vi "Dashboard Main.vi"() -> ()   [LabVIEW 2015]
uses:
  <vilib>/Utility/miscctls.llb/LVRowAndColumnTypeDef.ctl
  <vilib>/event_ctls.llb/eventvkey.ctl
  <vilib>/Rock Robotics/WPI/Dashboard/WPI_DashboardLogging Global.vi
  <vilib>/Rock Robotics/Network Tables/NT Read Numeric Array.vi
  <vilib>/Rock Robotics/Network Tables/NT Write String Array.vi
  <vilib>/Rock Robotics/Network Tables/NT Write Numeric Array.vi
  <vilib>/Utility/config.llb/Write Key (String).vi
  <vilib>/Utility/config.llb/Write Key (I32).vi
  <vilib>/Utility/config.llb/NI_LVConfig.lvlib
panel:
  in  "TCP":refnum<k5>
  in  "Rec Mode":enum32{"Stop", "Record", "Playback"}(radio)
  in  "Vision":u16(ring) items=["Camera Off", "USB Camera SW", "USB Camera HW", "IP Camera"]
  out "Camera IP":string
  out "Image Message":string="Timeout in Camera Communications"
  in  "Dashboard Tab":T1(tab)
  in  "Auto Routines":string(combo)
  out "NT Connected":bool
  in  "Camera Settings":T2={"Frame Rate"=30, "Compression"=30, "Size"=1} {"Frame Rate" scale=1.0..30.0; "Size" items=["640x480", "320x240", "160x120"]}
  out "MotorChart R":cluster{"Numeric":dbl, "Numeric":dbl}(graph)
  out "MotorChart L":T3(graph)
  out "MotorSliders R":cluster{"MotorSlide1":dbl, "MotorSlide2":dbl} {"MotorSlide2" scale=-1.0..1.0 scale format="%#_2e"; "MotorSlide1" scale=-1.0..1.0 scale format="%#_2e"}
  out "MotorSliders L":T4 {"MotorSlide4 2" scale=0.0..14.0 scale format="%#_2e"; "MotorSlide2" scale=-1.0..1.0 scale format="%#_2e"; "MotorSlide1" scale=-1.0..1.0 scale format="%#_2e"}
  out "Gyro":dbl(knob) scale=0.0..360.0
  out "JS1 Z":dbl(slide) scale=-1.0..1.0 scale format="%#_2e"
  out "JS1 Graph":cluster{"X":dbl, "Y":dbl}[](graph)
  out "JS1 Buttons":T5
  out "JS2 Z":dbl(slide) scale=-1.0..1.0 scale format="%#_2e"
  out "JS2 Graph":cluster{"X":dbl, "Y":dbl}[](graph)
  out "JS2 Buttons":T5
  out "Mode":T6(ring)=enum."Auto Disabled"
  in  "DB Camera Config":bool
  out "fps":dbl format="%#.1g"
  out "Mbps":dbl format="%#.1g"
  out "Mbps 2":bool
  in  "DB/String 9":string
  in  "DB/String 8":string
  in  "DB/String 7":string
  in  "DB/String 6":string
  in  "DB/String 5":string
  in  "DB/String 4":string
  in  "DB/String 3":string
  in  "DB/String 2":string
  in  "DB/String 1":string
  in  "DB/String 0":string
  in  "DB/Slider 0":dbl(slide) scale=0.0..5.0
  in  "DB/Slider 1":dbl(slide) scale=0.0..5.0
  in  "DB/Slider 2":dbl(slide) scale=0.0..5.0
  in  "DB/Slider 3":dbl(slide) scale=0.0..5.0
  out "DB/LED 3":bool
  out "DB/LED 2":bool
  out "DB/LED 1":bool
  out "DB/LED 0":bool
  in  "DB/Button 3":bool
  in  "DB/Button 2":bool
  in  "DB/Button 1":bool
  in  "DB/Button 0":bool caption="New Name"
  in  "Test Slider":dbl(slide) scale=0.0..100.0 scale format="%#_3g"
  in  "On/Off":bool caption="Solenoid"
  in  "Test Name":u16(ring) items=["Select the test to run..."]
  in  "Test Tree":string(tree)
  in  "Motor":cluster{"Value":dbl, "Enable":bool} {"Value" scale=-1.0..1.0 scale format="%#_3g"}
  out "Progress":T7 {"Test Progress" scale=0.0..100.0}
  in  "Rev/Fwd":cluster{"Forward":bool, "Reverse":bool}
  in  "Test Ring":u16(ring) items=["Monochrome", "Color"]
  out "Cmd Status":string
  in  "Execute Command":bool
  in  "Command Params":string[][](table)
  in  "Command Selection":i32(listbox)
  in  "CheckList":i32(listbox)
  out "Tree":string(tree)
  out "Camera Image":T8(plugin-control)
  out "Boolean":bool
  # "Left"
  # "Front"
  # "Right"
  # "Battery"
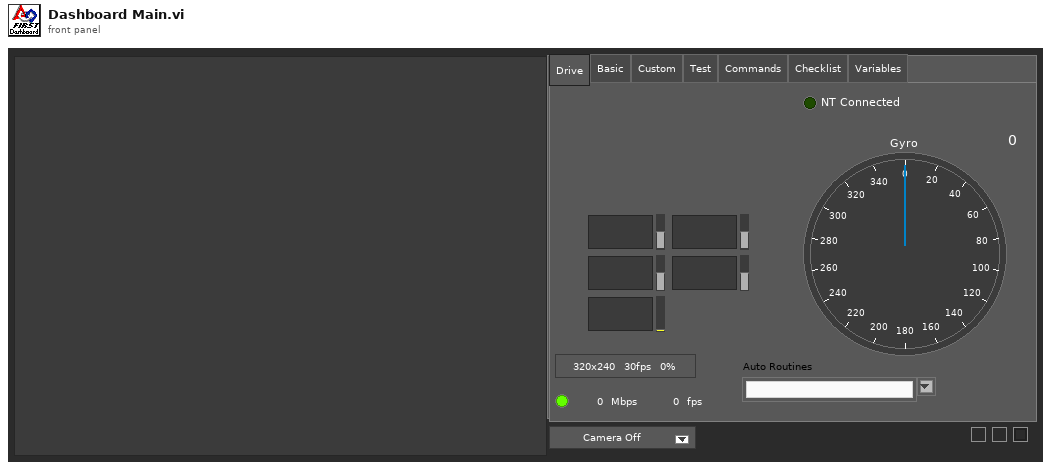
[diagram p1: front panel]
types:
  T1 = enum32{"Drive", "Basic", "Custom", "Test", "Commands", "Checklist", "Variables"}
  T2 = cluster{"Frame Rate":i32, "Compression":i32, "Size":u16}
  T3 = cluster{"Numeric":dbl, "Numeric":dbl, "Battery V":dbl}
  T4 = cluster{"MotorSlide1":dbl, "MotorSlide2":dbl, "MotorSlide4 2":dbl}
  T5 = cluster{bool, bool, bool, bool, bool, bool, bool, bool, bool, bool, bool, bool}
  T6 = enum8{"Tele-Op Disabled", "Tele-Op Enabled", "Auto Disabled", "Auto Enabled", "Test Disabled", "Test Enabled", "Disconnected", "No Code", "E-Stop"}
  T7 = cluster{"Test Progress":u8, "Test Progress Text":string}
  T8 = typedef "IMAQ Image.ctl" = refnum<image>
  T9 = cluster{"IDs":cluster{"RPC field ID":u16, "Unique ID":u16}, "String":string}
  T10 = enum32{"Drive", "Basic", "Custom", "Test", "Checklist", "Variables"}
  T11 = typedef "Image Type" = u32
  T12 = cluster{"Camera Image":refnum<vi>, "Dashboard Tab":refnum<vi>, "Boolean":refnum<vi>, "Vision":refnum<vi>, "Rec Mode":refnum<vi>, "Test Slider":refnum<vi>, "On/Off ":refnum<vi>, "Test Ring":refnum<vi>, "Rev/Fwd":refnum<vi>, "Test Name":refnum<vi>, "Motor":refnum<vi>, "Progress":refnum<vi>, "CheckList":refnum<vi>, "Tree":refnum<vi>, "Test Tree":refnum<vi>, "Command Params":refnum<vi>, "Command Selection":refnum<vi>, "Execute Command":refnum<vi>, "Cmd Status":refnum<vi>}
  T13 = cluster{"Error Strings":string, "Disable Counts":cluster{u16, u16}, "Rail Faults":cluster{u16, u16, u16}, "Robot IP":string, "DB Mode":u8, "Event Info":cluster{"Name":string, "Type":u8, "Number":u16, "Replay":u8}, "Camera Addr":string}
  T14 = cluster{"Storage":cluster{"Disk Free":u64, "RAM Block":u32, "RAM free":u32}, "CPU Utilization":cluster{"CPU % ISR":sgl, "CPU % Time Crit":sgl, "CPU % Timed Str":sgl, "CPU % High":sgl, "CPU % Above":sgl, "CPU % Normal":sgl, "CPU % Low":sgl}, "CAN":cluster{"% Bus Utilization":sgl, "Bus Off Cnt":u32, "TX_FIFO Full Cnt":u32, "Receive Error Cnt":u8, "Transmit Error Cnt":u8}, "HID":cluster{"HID Outputs":u32, "Rumble Low":u16, "Rumble High":u16}[]}
  T15 = cluster{"Status bits":cluster{"Test Mode":bool, "Autonomous":bool, "Enabled":bool, "Code Start":bool, "Brownout":bool, "Reserved 2":bool, "Reserved 3":bool, "E-Stop":bool}, "Code Trace":cluster{"Disabled":bool, "TeleOp":bool, "Auto":bool, "Test":bool}, "Controller Type":enum16{"unknown", "cRIO", "roboRio"}, "Code?":enum16{"unknown", "noCode", "code"}, "Battery V":dbl}
  T16 = cluster{"Control Bits":cluster{"TestMode":bool, "Autonomous":bool, "Enabled":bool, "FMS Present":bool, bool, bool, bool, "E-Stop":bool}, "Team Station ":u8, "Countdown":sgl, "Joystick Values":cluster{"Axes":dbl[], "Buttons":bool[], "POVs":i16[]}[]}
  T17 = cluster{"Axes":dbl[], "Buttons":bool[], "POVs":i16[]}[]
  T18 = cluster{"Axes":dbl[], "Buttons":bool[], "POVs":i16[]}
  T19 = cluster{"Buttons[0]":bool, "Buttons[1]":bool, "Buttons[2]":bool, "Buttons[3]":bool, "Buttons[4]":bool, "Buttons[5]":bool, "Buttons[6]":bool, "Buttons[7]":bool, "Buttons[8]":bool, "Buttons[9]":bool, "Buttons[10]":bool, "Buttons[11]":bool}
  T20 = typedef "NI_LVConfig.lvlib/Config Data RefNum.ctl" = refnum<k1>
  T21 = cluster{"Operation":enum16{"Update", "Clear"}, "Color Box":u32}[]
  T22 = typedef "eventvkey.ctl" = enum16{"ASCII", "Enter", "Return", "Shift", "Ctrl", "Alt", "Cmd", "Opt", "Caps", "NumLock", "Clear", "Break", "Up", "Down", "Left", "Right", "Insert", "Delete", "Home", "End", "PageUp", "PageDown", "Escape", "Help", "Pause", "ScrollLock", "F1", "F2", "F3", "F4", "F5", "F6", "F7", "F8", "F9", "F10", "F11", "F12", "F13", "F14", "F15", "F16", "F17", "F18", "F19", "F20", "F21", "F22", "F23", "F24", "Play", "VolumeUp", "VolumeDown", "Mute", "Two Byte Char"}
  T23 = cluster{"Image Size":bool, "Image Type":bool, "Pixel Value":bool, "ROI Information":bool, "Zoom Factor":bool}
  T24 = enum8{"Enabled", "Disabled", "Disabled and Grayed Out"}
  T25 = cluster{"Operation":enum16{"Update", "Clear"}, "Color Box":u32}
  T26 = typedef "LVRowAndColumnTypeDef.ctl" = cluster{"Row":i32, "Column":i32}
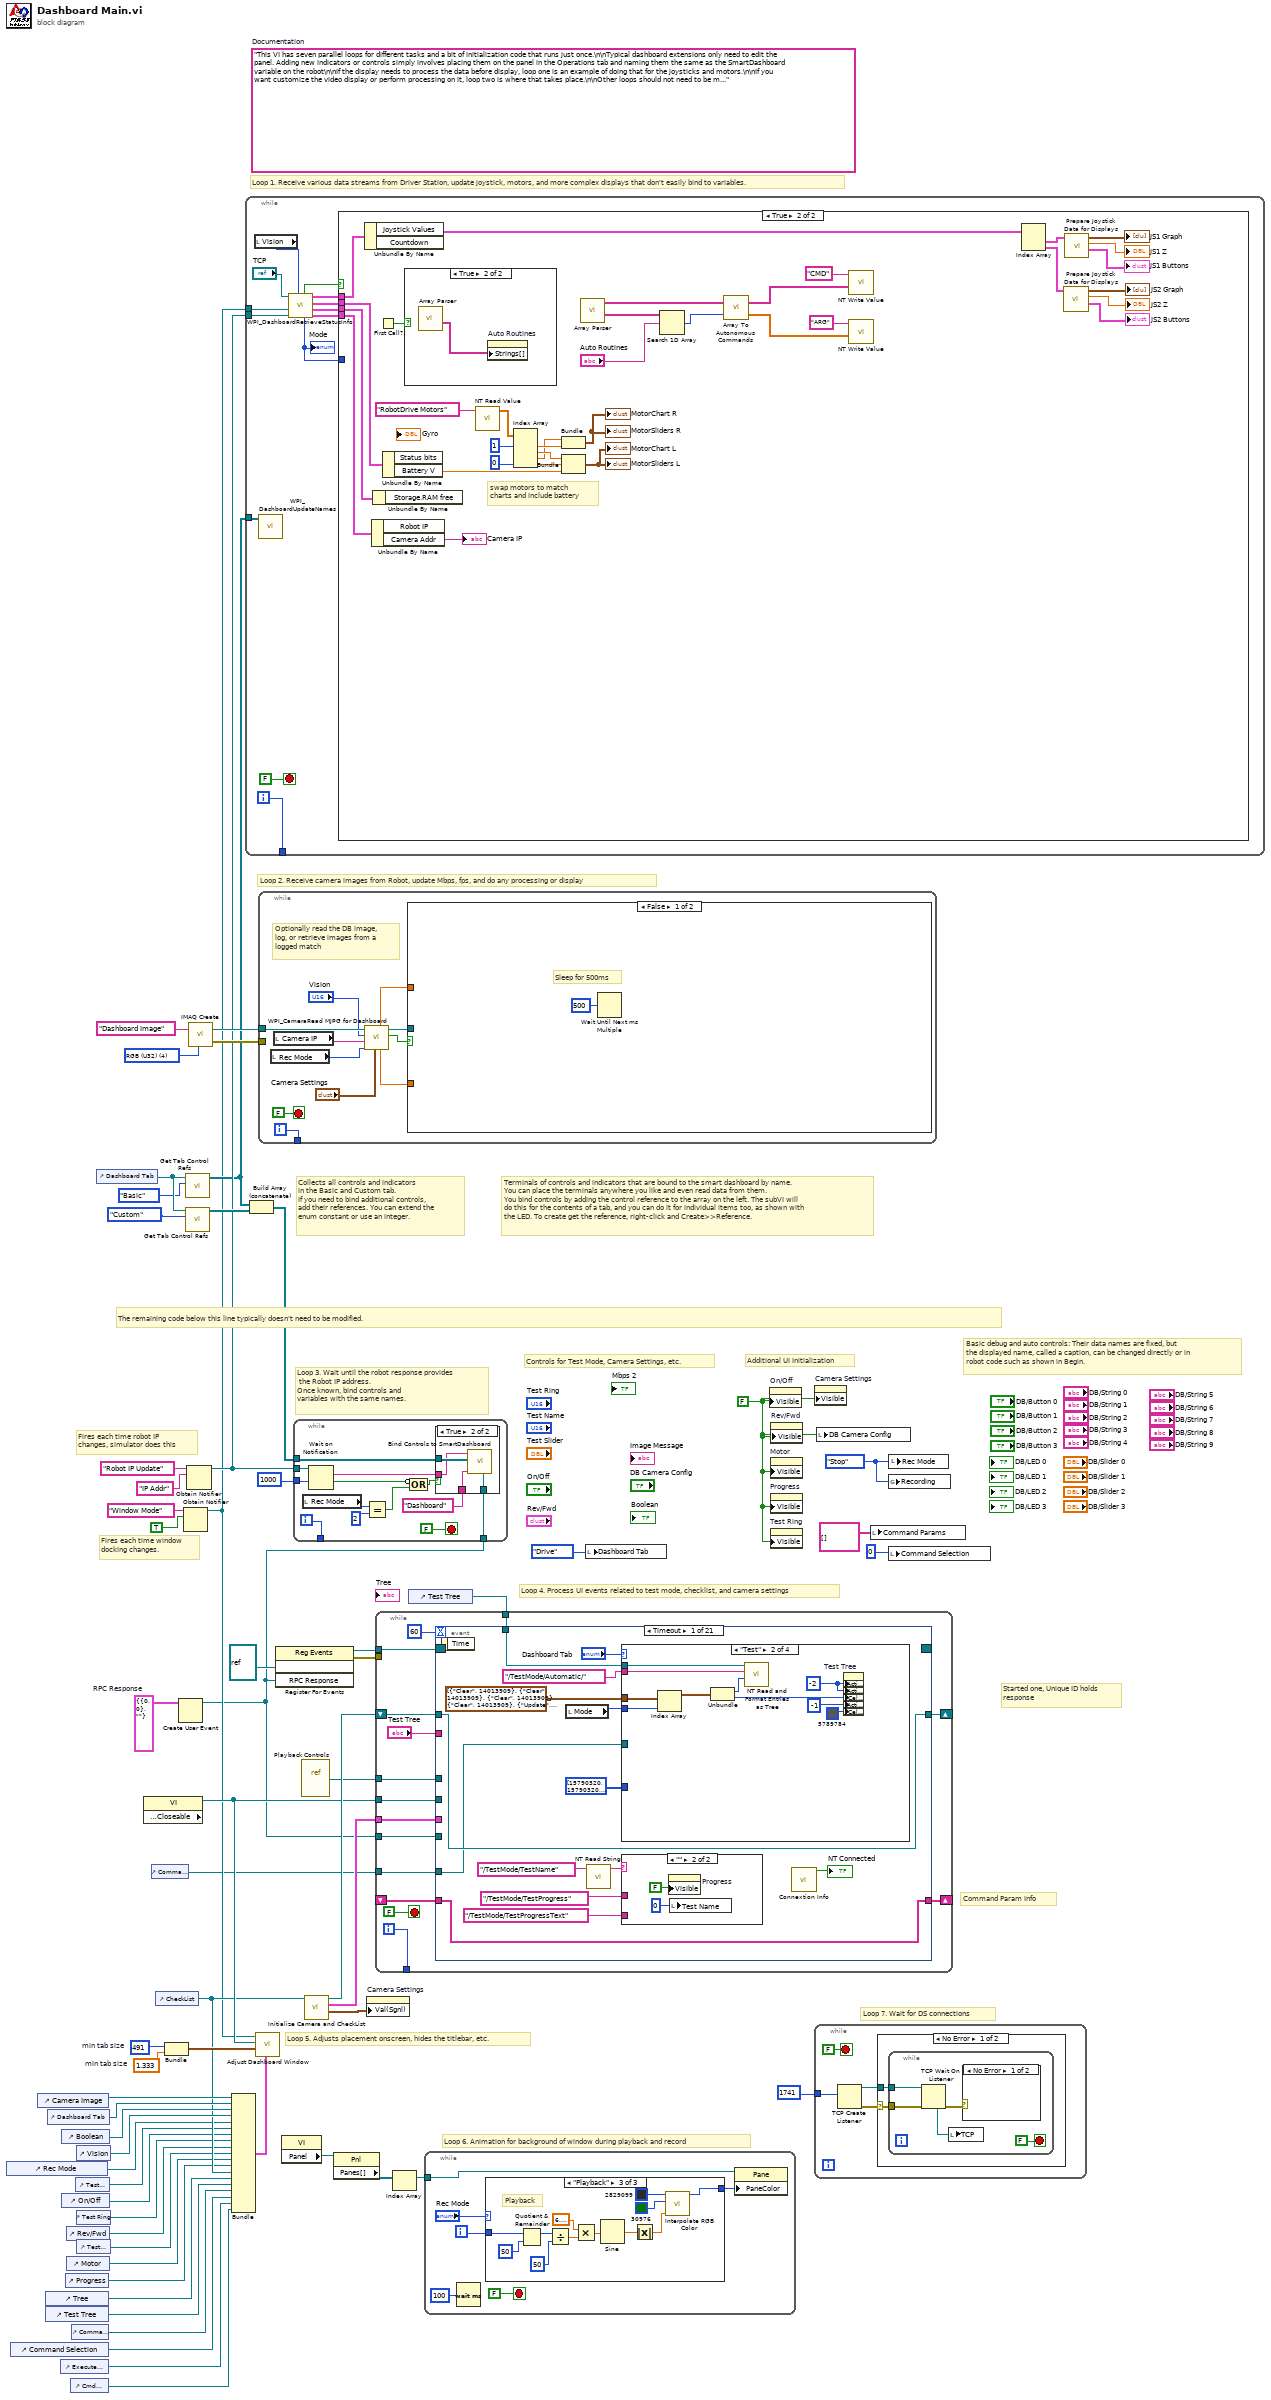
[diagram p0: block diagram]
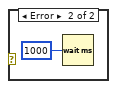
[diagram p2: hidden frame]
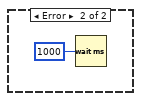
[diagram p3: hidden frame]
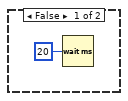
[diagram p4: hidden frame]
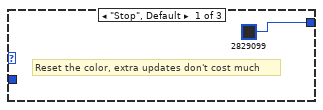
[diagram p6: hidden frame]
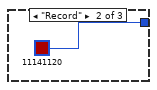
[diagram p7: hidden frame]
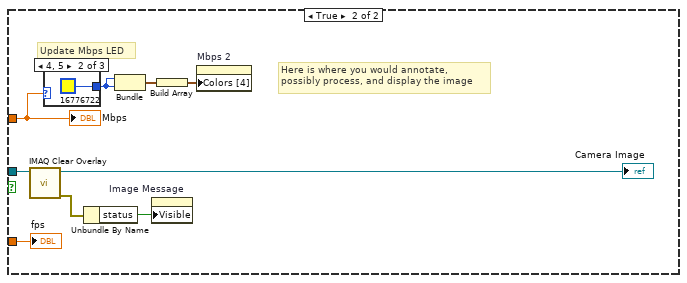
[diagram p9: hidden frame]
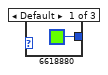
[diagram p10: hidden frame]
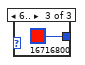
[diagram p11: hidden frame]
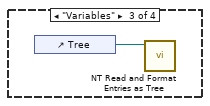
[diagram p13: hidden frame]
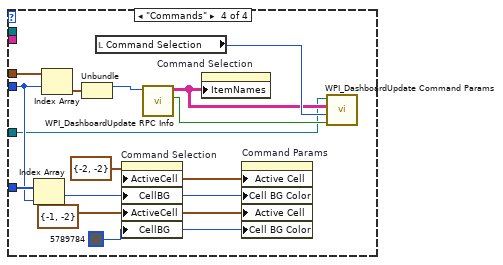
[diagram p14: hidden frame]
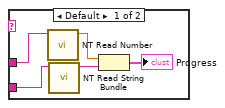
[diagram p15: hidden frame]
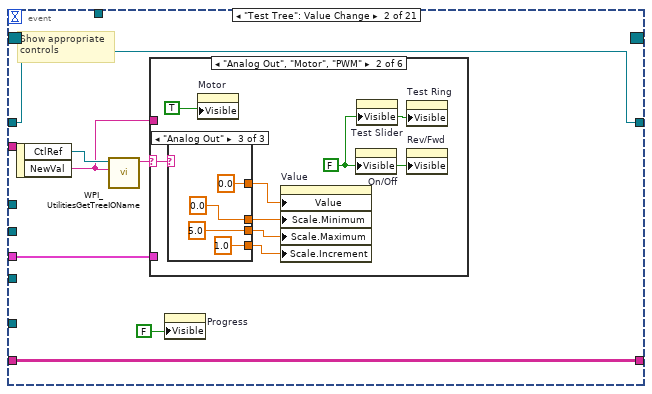
[diagram p16: hidden frame]
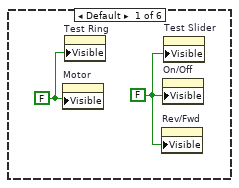
[diagram p17: hidden frame]
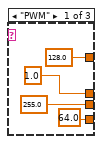
[diagram p18: hidden frame]
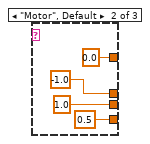
[diagram p19: hidden frame]
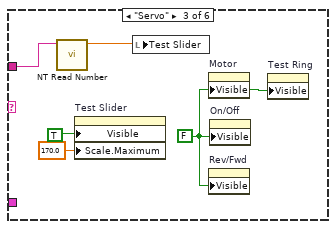
[diagram p20: hidden frame]
diagram:
  w7 = T9 {"IDs"={"RPC field ID"=0, "Unique ID"=0}, "String"=""}  # RPC Response
  w33 = 491  # min tab size
  w32 = 1.333  # min tab size
  w41 = enum32{"Stop", "Record", "Playback"}."Stop" ("Rec Mode")
  w15 = FALSE ("Visible")
  (unwired) "This VI has seven parallel loops for different tasks and a bit of initialization code that runs just once.\n\nTypical dashboard extensions only need to edit the panel. Adding new indicators or controls simply involves placing them on the panel in the Operations tab and naming them the same as the SmartDashboard variable on the robot\n\nIf the display needs to process the data before display, loop one is an example of doing that for the joysticks and motors.\n\nIf you want customize the video display or perform processing on it, loop two is where that takes place.\n\nOther loops should not need to be modified. They are pretty standard, and document the task they perform."  # Documentation
  w61 = T11 4 items=["Grayscale (U8)", "Grayscale (I16)", "Grayscale (SGL)", "Complex (CSG)", "RGB (U32)", "HSL (U32)", "RGB (U64)"] ("Image Type")
  # "Command Param Info"
  # "Started one, Unique ID holds\nresponse"
  # "Loop 7. Wait for DS connections"
  # "Basic debug and auto controls: Their data names are fixed, but\nthe displayed name, called a caption, can be changed directly or in\nrobot code such as shown in Begin."
  # "Controls for Test Mode, Camera Settings, etc."
  # "Additional UI Initialization"
  # "Loop 6. Animation for background of window during playback and record"
  # "Fires each time robot IP\nchanges, simulator does this"
  # "Fires each time window\ndocking changes."
  # "Collects all controls and indicators\nin the Basic and Custom tab.\nIf you need to bind additional controls,\nadd their references. You can extend the\nenum constant or use an integer."
  # "The remaining code below this line typically doesn't need to be modified."
  # "Loop 4. Process UI events related to test mode, checklist, and camera settings"
  # "Terminals of controls and indicators that are bound to the smart dashboard by name.\nYou can place the terminals anywhere you like and even read data from them.\nYou bind controls by adding the control reference to the array on the left. The subVI will\ndo this for the contents of a tab, and you can do it for individual items too, as shown with\nthe LED. To create get the reference, right-click and Create>>Reference."
  # "Loop 3. Wait until the robot response provides\n the Robot IP address.\nOnce known, bind controls and\nvariables with the same names."
  # "Loop 5. Adjusts placement onscreen, hides the titlebar, etc."
  # "Loop 1. Receive various data streams from Driver Station, update joystick, motors, and more complex displays that don't easily bind to variables."
  # "Loop 2. Receive camera images from Robot, update Mbps, fps, and do any processing or display"
  n1 = control-ref of="Rec Mode"() -> (w21:refnum<vi>)
  n2 = control-ref of="Command Selection"() -> (w6:refnum<vi>)
  n3 = control-ref of="Camera Image"() -> (w36:refnum<vi>)
  n4 = control-ref of="Tree"() -> (w25:refnum<vi>)
  n5 = control-ref of="Test Tree"() -> (w24:refnum<vi>)
  n6 = control-ref of="Dashboard Tab"() -> (w35:refnum<vi>)
  n7 = control-ref of="Execute Command"() -> (w8:refnum<vi>)
  n8 = control-ref of="Boolean"() -> (w30:refnum<vi>)
  n9 = control-ref of="On/Off"() -> (w19:refnum<vi>)
  n10 = control-ref of="Progress"() -> (w16:refnum<vi>)
  n11 = control-ref of="Rev/Fwd"() -> (w17:refnum<vi>)
  n12 = control-ref of="Motor"() -> (w22:refnum<vi>)
  n13 = control-ref of="Cmd Status"() -> (w2:refnum<vi>)
  n14 = control-ref of="Command Params"() -> (w9:refnum<vi>)
  n15 = control-ref of="Test Slider"() -> (w20:refnum<vi>)
  n16 = control-ref of="Vision"() -> (w34:refnum<vi>)
  n17 = control-ref of="Test Ring"() -> (w18:refnum<vi>)
  n18 = control-ref of="Test Name"() -> (w23:refnum<vi>)
  n19 = control-ref of="Dashboard Tab"() -> (w39:refnum<vi>)
  n20 = property class="VI" props=["Front Panel.Closeable"]() -> (reference out=w40:refnum<vi>)  [unwired: 2 in, 2 out]
  n21 = control-ref of="Command Params"() -> (w1:refnum<vi>)
  n22 = control-ref of="CheckList"() -> (w26:refnum<vi>)
  n23 = Bundle("min tab size"=w33, "min tab size"=w32) -> (w31:cluster{"min tab size":i32, "min tab size":dbl})  [unwired: 1 in]
  n24 = Create User Event(user event datatype=w7) -> (user event=w3:refnum<user-event>)  [unwired: 1 in, 1 out]
  n25 = Obtain Notifier(name (unnamed)="Window Mode", notification data type=TRUE) -> (notifier out=w12:refnum<notifier>)  [unwired: 2 in, 2 out]
  n26 = call <vilib>:"Get Tab Control Refs.vi"("Page Index"=T10."Basic" ("Dashboard Tab"), "TabControl in"=w39) -> ("ControlsOnPage"=w13:refnum<vi>[])  [unwired: 9 in]
  n27 = call <vilib>:"Get Tab Control Refs.vi"("Page Index"=T10."Custom" ("Dashboard Tab"), "TabControl in"=w39) -> ("ControlsOnPage"=w38:refnum<vi>[])  [unwired: 9 in]
  n28 = Obtain Notifier(name (unnamed)="Robot IP Update", notification data type="IP Addr" ("name (unnamed)")) -> (notifier out=w14:refnum<notifier>)  [unwired: 2 in, 2 out]
  n29 = call "IMAQ Create"("Image Name"="Dashboard Image", "Image Type"=w61) -> ("New Image"=w59:T8, "error out"=w58:errorcluster)  [unwired: 2 in, 1 out]
  n30 = Bundle("Camera Image"=w36, "Dashboard Tab"=w35, "Boolean"=w30, "Vision"=w34, "Rec Mode"=w21, "Test Slider"=w20, "On/Off"=w19, "Test Ring"=w18, "Rev/Fwd"=w17, "Test Name"=w23, "Motor"=w22, "Progress"=w16, "CheckList"=w26, "Tree"=w25, "Test Tree"=w24, "Command Params"=w9, "Command Selection"=w6, "Execute Command"=w8, "Cmd Status"=w2) -> (w27:T12)  [unwired: 1 in]
  n31 = while {
    tunnel: [w73] -> _
    tunnel: w14 -> [w67]
    tunnel: w13 -> [w66]
    tunnel: w12 -> [w62]
    i -> [w73]
    stop <- FALSE stop-if-true
    n32 = local read "Vision"() -> (w64:u16)
    n33 = call <vilib>:"WPI_DashboardUpdateNames.vi"("Controls on Tab"=w66) -> ()  [unwired: 11 in]
    n34 = call <vilib>:"WPI_DashboardRetrieveStatusInfo.vi"("Vision"=w64, "Binding Refnum"=w67, "Window Mode Notifier"=w62, "TCP Cnx"="TCP") -> ("Power and Errors"=w68:T13, "Robot Metrics"=w71:T14, "Status Info"=w72:T15, "Control Info"=w69:T16, "Robot Mode"=w65:T6, "Process?"=w70:bool)  [unwired: 2 in]
    "Mode" <- w65
    n35 = case shown="True" w70 {
      tunnel: w72 -> [_ w109]
      tunnel: w71 -> [_ w108]
      tunnel: w69 -> [_ w107]
      tunnel: w68 -> [_ w106]
      tunnel: w65 -> [_ _]
      frame False {
        n36 = Wait (ms)(milliseconds to wait=u32 20) -> ()  [unwired: 1 out]
      }
      frame True {
        # "swap motors to match\ncharts and include battery"
        n37 = Unbundle By Name(w107) -> ("Joystick Values"=w96:T17)  [unwired: 1 out]
        n38 = Unbundle By Name(w106) -> ("Camera Addr"=→"Camera IP":string)  [unwired: 1 out]
        n39 = Unbundle By Name(w108) -> ()  [unwired: 1 out]
        n40 = First Call?() -> (First Call?: T/F=w76:bool)
        n41 = Unbundle By Name(w109) -> ("Battery V"=w97:dbl)  [unwired: 1 out]
        n42 = case shown="True" w76 {
          frame False {
          }
          frame True {
            n43 = call "Array Parser.vi"() -> ("Auto Routines"=w110:string[])  [unwired: 9 in, 2 out]
            n44 = property on="Auto Routines" class="CmbBox"("Strings[]"=w110) -> ()  [unwired: 2 in, 2 out]
          }
        }
        n45 = call-poly <vilib>:"NT Read Value.vi"("Name"="RobotDrive Motors") -> ("Numeric Array"=w85:dbl[])  [unwired: 9 in, 1 out]
        n46 = Index Array(array=w85, index #1=1, index #4=0) -> (element #1=w101:dbl, element #2=w102:dbl, element #3=w100:dbl, element #4=w105:dbl)  [unwired: 2 in]
        n47 = Bundle("Numeric"=w100, "Numeric"=w101) -> (→"MotorChart R" →"MotorSliders R":cluster{"Numeric":dbl, "Numeric":dbl})  [unwired: 1 in]
        n48 = Bundle("Numeric"=w102, "Numeric"=w105, "Battery V"=w97) -> (→"MotorChart L" →"MotorSliders L":T3)  [unwired: 1 in]
        n49 = call "Array Parser.vi"() -> ("Auto Routines"=w79:string[], "CSV Data"=w77:string[][][])  [unwired: 9 in, 1 out]
        n50 = Search 1D Array(1D array=w79, element="Auto Routines") -> (index of element=w78:i32)  [unwired: 1 in]
        n51 = call "Array To Autonomous Commands.vi"("Which"=w78, "Input Array"=w77) -> ("Float Output Array"=w81:dbl[], "String Output Array"=w82:string[])
        n52 = call-poly <vilib>:"NT Write Value.vi"("String Array"=w82, "Name"="CMD") -> ()  [unwired: 9 in, 1 out]
        n53 = call-poly <vilib>:"NT Write Value.vi"("Numeric Array"=w81, "Name"="ARG") -> ()  [unwired: 9 in, 1 out]
        n54 = Index Array(array=w96) -> (element #1=w95:T18, element #2=w90:T18)  [unwired: 2 in]
        n55 = call "Prepare Joystick Data for Displays.vi"("Joystick Values"=w90) -> ("Buttons"=→"JS2 Buttons":T19, "Z Axis"=→"JS2 Z":dbl, "Cartesian Data"=→"JS2 Graph":cluster{"X axis":dbl, "X axis":dbl}[])  [unwired: 8 in]
        n56 = call "Prepare Joystick Data for Displays.vi"("Joystick Values"=w95) -> ("Buttons"=→"JS1 Buttons":T19, "Z Axis"=→"JS1 Z":dbl, "Cartesian Data"=→"JS1 Graph":cluster{"X axis":dbl, "X axis":dbl}[])  [unwired: 8 in]
      }
    }
  }
  n57 = Build Array (concatenate)(w13, w38) -> (w37:refnum<vi>[])
  n58 = call "Adjust Dashboard Window.vi"("Sizing Refnums"=w27, "Size Constraints"=w31, "VI"=w40, "WIn Mode"=w12) -> ()  [unwired: 8 in]
  n59 = while {
    tunnel: w59 -> [w119]
    tunnel: w58 -> [_]
    tunnel: [w120] -> _
    i -> [w120]
    stop <- FALSE stop-if-true
    # "Optionally read the DB image,\nlog, or retrieve images from a\nlogged match"
    n60 = local read "Rec Mode"() -> (w113:enum32{"Stop", "Record", "Playback"})
    n61 = local read "Camera IP"() -> (w111:string)
    n62 = call <vilib>:"WPI_CameraRead MJPG for Dashboard.vi"("Camera Settings"="Camera Settings", "Rec Mode"=w113, "Camera IP"=w111, "Camera Mode"="Vision", "Refnum in"=w119) -> ("Active"=w117:bool, "Refnum out"=w118:T8, "FPS"=w116:dbl, "Bandwidth (Mbps)"=w115:dbl)  [unwired: 3 in]
    n63 = case shown="False" w117 {
      tunnel: w118 -> [_ w126]
      tunnel: w115 -> [_ w125]
      tunnel: w116 -> [_ w123]
      frame False {
        # "Sleep for 500ms"
        n64 = Wait Until Next ms Multiple(millisecond multiple=u32 500) -> ()  [unwired: 1 out]
      }
      frame True {
        # "Here is where you would annotate,\npossibly process, and display the image"
        # "Update Mbps LED"
        n65 = call "IMAQ Clear Overlay"("Image"=w126) -> ("error out"=w130:errorcluster, "Image Out"=→"Camera Image":T8)  [unwired: 2 in, 7 out]
        n66 = case shown="4, 5" w125 {
          tunnel: [u32 6618880 ("Color Box") u32 16776722 ("Color Box") u32 16716800 ("Color Box")] -> w127
          frame Default {
          }
          frame 4, 5 {
          }
          frame 6.. {
          }
        }
        n67 = Unbundle By Name(w130) -> ("status"=w131:bool)
        n68 = Bundle("Color Box"=w127, "Color Box"=w127) -> (w129:cluster{"Color Box":u32, "Color Box":u32})  [unwired: 1 out]
        n69 = property on="Image Message" class="Str"("Visible"=w131) -> ()  [unwired: 2 in, 2 out]
        n70 = Build Array(w129) -> (w128:cluster{"Color Box":u32, "Color Box":u32}[])
        n71 = property on="Mbps 2" class="Bool (strict)"("Colors [4]"=w128) -> ()  [unwired: 2 in, 2 out]
        "Mbps" <- w125
        "fps" <- w123
      }
    }
  }
  n72 = register-events(refnum<vi> refnum, w3) -> (reference out=w45:refnum<event-registration>, error out=w44:errorcluster)  [unwired: 2 in]
  n73 = property class="VI"() -> ("Panel"=w48:refnum<vi>)  [unwired: 2 in, 2 out]
  n74 = while {
    tunnel: w37 -> [w147]
    tunnel: w14 -> [w145]
    tunnel: [w143] -> _
    tunnel: u32 1000 ("milliseconds to wait") -> [w142]
    tunnel: w3 -> [w135]
    i -> [w143]
    stop <- FALSE stop-if-true
    n75 = local read "Rec Mode"() -> (w138:enum32{"Stop", "Record", "Playback"})
    n76 = Wait on Notification(notifier=w145, timeout in ms (-1)=w142) -> (notification=w144:string, timed out?=w140:bool)  [unwired: 2 in, 2 out]
    n77 = Equal?(x=w138, y=u16 2 ("Rec Mode")) -> (x = y?=w139:bool)
    n78 = Compound Arithmetic op=OR(invert w140, w139) -> (w141:bool)
    n79 = case shown="True" w141 {
      tunnel: w147 -> [_ w151]
      tunnel: w144 -> [_ w150]
      tunnel: "Dashboard" -> [_ w149]
      tunnel: w135 -> [_ w148]
      frame False {
      }
      frame True {
        n80 = call <vilib>:"Bind Controls to SmartDashboard.vi"("RPC ref"=w148, "Client Name"=w149, "Bound Control Refs"=w151, "Server IP Address"=w150) -> ()  [unwired: 8 in]
      }
    }
  }
  n81 = vi-ref "Playback Controls.vi"() -> (w46:refnum<vi>)
  n82 = call "Initialize Camera and CheckList.vi"("ListBox in"=w26) -> ("Cluster"=w52:cluster{"value":i32, "value":i32, "index":i32}, "Array"=w53:cluster{string[]}[], "File Refnum"=w51:T20)  [unwired: 8 in]
  n83 = property class="Pnl"(reference=w48) -> ("Panes[]"=w49:refnum<vi>[])  [unwired: 1 in, 2 out]
  n84 = property on="Camera Settings" class="Clust (strict)"("Val(Sgnl)"=w52) -> ()  [unwired: 2 in, 2 out]
  n85 = Index Array(array=w49) -> (element=w47:refnum<vi>)  [unwired: 1 in]
  n86 = control-ref of="Test Tree"() -> (w50:refnum<vi>)
  n87 = while {
    tunnel: w53 -> [w163]
    shift-right: [w162] -> _
    shift-left: w51 -> [w161]
    tunnel: [w160] -> _
    tunnel: w50 -> [w159]
    tunnel: w46 -> [w158]
    tunnel: w45 -> [w157]
    tunnel: w44 -> [_]
    tunnel: w40 -> [w156]
    tunnel: w3 -> [w155]
    tunnel: w1 -> [w154]
    shift-right: [w153] -> _
    shift-left: _ -> [w152]
    i -> [w160]
    stop <- FALSE stop-if-true
    n88 = event shown="[0] Timeout" {
      selector: w157 -> [_ _ _ _ _ _ _ _ _ _ _ _ _ _ _ _ _ _ _ _ _]
      dyn-events: [_ _ _ _ _ _ _ _ _ _ _ _ _ _ _ _ w464 _ _ _ _] -> _
      timeout: u32 60 ("milliseconds to wait") -> [_ _ _ _ _ _ _ _ _ _ _ _ _ _ _ _ _ _ _ _ _]
      tunnel: w159 -> [w176 _ _ _ _ _ _ _ _ _ _ _ _ _ _ _ _ _ _ _ _]
      tunnel: "Test Tree" -> [_ _ _ _ _ _ _ _ _ _ _ w427 w436 w439 w444 w453 _ _ _ _ _]
      tunnel: w163 -> [_ w214 _ _ _ _ _ _ _ w389 w420 _ _ _ _ _ _ _ _ _ _]
      tunnel: [w173 w213 w317 w323 w335 w347 w355 w361 w374 w388 w413 w426 w434 w438 w443 w452 w466 w482 w484 w492 w503] -> w162
      tunnel: w161 -> [w173 w213 w317 w323 w335 w347 w355 w361 w374 w387 w413 w426 w434 w438 w443 w452 w466 w482 w484 w492 w503]
      tunnel: w158 -> [_ _ _ _ _ _ _ _ _ _ _ _ _ _ _ _ w467 _ w487 _ _]
      tunnel: w156 -> [_ _ _ _ _ _ _ _ _ _ _ _ _ _ _ _ w462 _ _ _ _]
      tunnel: w155 -> [_ _ _ _ _ _ _ _ _ _ _ _ _ _ _ _ w458 _ _ _ _]
      tunnel: w154 -> [w168 _ _ _ w333 _ _ _ _ _ _ _ _ _ _ _ _ _ _ _ _]
      tunnel: [w167 w212 w316 w322 w331 w341 w352 w360 w373 w386 w412 w425 w433 w437 w442 w451 w457 w480 w483 w488 w496] -> w153
      tunnel: w152 -> [w167 w212 w316 w322 w331 _ _ w360 w373 w386 w412 w425 w433 w437 w442 w451 w457 w480 w483 w488 w496]
      event Timeout {
        n89 = event-data() -> ()  [unwired: 1 in, 1 out]
        n90 = local read "Mode"() -> (w170:T6)
        n91 = call <vilib>:"NT Read String.vi"("Name"="/TestMode/TestName") -> ("String"=w179:string)  [unwired: 9 in, 1 out]
        n92 = case shown="\"Test\"" "Dashboard Tab" {
          tunnel: w176 -> [_ w190 _ _]
          tunnel: "/TestMode/Automatic/" ("Name Pattern") -> [_ w189 _ _]
          tunnel: T21 [{"Operation"=enum."Clear", "Color Box"=14013909}, {"Operation"=enum."Clear", "Color Box"=14013909}, {"Operation"=enum."Clear", "Color Box"=14013909}, {"Operation"=enum."Clear", "Color Box"=14013909}, {"Operation"=enum."Update", "Color Box"=14013909}, {"Operation"=enum."Update", "Color Box"=16777215}, {"Operation"=enum."Clear", "Color Box"=14013909}, {"Operation"=enum."Clear", "Color Box"=14013909}, {"Operation"=enum."Clear", "Color Box"=14013909}] -> [_ w182 _ w199]
          tunnel: w170 -> [_ w181 _ w198]
          tunnel: u32[] [15790320, 15790320, 15790320, 15790320, 16777215, 16777215, 15790320, 15790320, 15790320] -> [_ _ _ w204]
          tunnel: w168 -> [_ _ _ w192]
          frame "Custom", Default {
          }
          frame "Test" {
            w188 = -2 ("Active Item:Row Number")
            n93 = Index Array(array=w182, index=w181) -> (element=w183:T25)
            n94 = Unbundle(w183) -> ("Operation"=w184:enum16{"Update", "Clear"}, "Color Box"=w185:u32)
            n95 = call <vilib>:"NT Read and Format Entries as Tree.vi"("Operation"=w184, "Name Pattern"=w189, "Tree Refnum"=w190) -> ()  [unwired: 7 in, 2 out]
            n96 = property on="Test Tree" class="Tree (strict)"("Active Item Row Number"=w188, "ActiveColNum"=w188, "CellBG"=w185, "Active Item Row Number"=-1 ("Active Item:Row Number"), "CellBG"=u32 5789784 ("Color Box")) -> ()  [unwired: 2 in, 2 out]
          }
          frame "Variables" {
            n97 = control-ref of="Tree"() -> (w191:refnum<vi>)
            n98 = call <vilib>:"NT Read and Format Entries as Tree.vi"("Tree Refnum"=w191) -> ()  [unwired: 9 in, 2 out]
          }
          frame "Commands" {
            w200 = u32 5789784 ("Color Box")
            w201 = T26 {"Row"=-1, "Column"=-2} ("Active Cell:Active Cell")
            w203 = T26 {"Row"=-2, "Column"=-2} ("Active Cell:Active Cell")
            n99 = Index Array(array=w204, index=w198) -> (element=w202:u32)
            n100 = Index Array(array=w199, index=w198) -> (element=w197:T25)
            n101 = Unbundle(w197) -> ("Operation"=w196:enum16{"Update", "Clear"})  [unwired: 1 out]
            n102 = local read "Command Selection"() -> (w195:i32)
            n103 = property on="Command Selection" class="MCListbox (strict)"("ActiveCell"=w203, "CellBG"=w202, "ActiveCell"=w201, "CellBG"=w200) -> ()  [unwired: 2 in, 2 out]
            n104 = call <vilib>:"WPI_DashboardUpdate RPC Info.vi"("Operation"=w196) -> ("update"=w194:bool, "commands"=w193:string[][])  [unwired: 9 in]
            n105 = property on="Command Selection" class="MCListbox (strict)"("ItemNames"=w193) -> ()  [unwired: 2 in, 2 out]
            n106 = property on="Command Params" class="Tbl (strict)"("Active Cell"=w203, "Cell BG Color"=w202, "Active Cell"=w201, "Cell BG Color"=w200) -> ()  [unwired: 2 in, 2 out]
            n107 = call <vilib>:"WPI_DashboardUpdate Command Params.vi"("Update"=w194, "NewVal"=w195, "Commands"=w193, "Param Tbl"=w192) -> ()  [unwired: 7 in, 1 out]
          }
        }
        n108 = case shown="\"\"" w179 {
          tunnel: "/TestMode/TestProgress" ("Name") -> [w206 _]
          tunnel: "/TestMode/TestProgressText" ("Name") -> [w205 _]
          frame Default {
            n109 = call <vilib>:"NT Read Number.vi"("Name"=w206) -> ("Numeric"=w207:dbl)  [unwired: 9 in, 1 out]
            n110 = call <vilib>:"NT Read String.vi"("Name"=w205) -> ("String"=w208:string)  [unwired: 9 in, 1 out]
            n111 = Bundle("Numeric"=w207, "String"=w208) -> (→"Progress":cluster{"Numeric":dbl, "String":string})  [unwired: 1 in]
          }
          frame "" {
            n112 = property on="Progress" class="Clust (strict)"("Visible"=FALSE) -> ()  [unwired: 2 in, 2 out]
            n113 = local write "Test Name"(u16 0) -> ()
          }
        }
        n114 = call <vilib>:"Connextion Info.vi"() -> ("Connected"=→"NT Connected":bool)  [unwired: 10 in, 1 out]
      }
      event "Test Tree": Value Change {
        # "Show appropriate\ncontrols"
        n115 = event-data() -> ("CtlRef"=w217:refnum<vi>, "NewVal"=w215:string)  [unwired: 1 in]
        n116 = call <vilib>:"WPI_UtilitiesGetTreeIOName.vi"("NewVal"=w215, "TreeControl in"=w217) -> ("I/O Name"=w218:string)  [unwired: 9 in]
        n117 = case shown="\"Analog Out\", \"Motor\", \"PWM\"" w218 {
          selector: w218 -> [_ w225 _ w247 w256 _]
          tunnel: w215 -> [_ _ w244 w246 _ w263]
          tunnel: w214 -> [_ _ _ _ _ w262]
          frame Default {
            w220 = FALSE ("Visible")
            w219 = FALSE ("Visible")
            n118 = property on="Motor" class="Clust (strict)"("Visible"=w219) -> ()  [unwired: 2 in, 2 out]
            n119 = property on="Test Ring" class="Ring (strict)"("Visible"=w219) -> ()  [unwired: 2 in, 2 out]
            n120 = property on="Rev/Fwd" class="Clust (strict)"("Visible"=w220) -> ()  [unwired: 2 in, 2 out]
            n121 = property on="On/Off" class="Bool (strict)"("Visible"=w220) -> ()  [unwired: 2 in, 2 out]
            n122 = property on="Test Slider" class="Slide (strict)"("Visible"=w220) -> ()  [unwired: 2 in, 2 out]
          }
          frame "Analog Out", "Motor", "PWM" {
            w226 = FALSE ("Visible")
            n123 = case shown="\"Analog Out\"" w225 {
              tunnel: [1.0 ("Value") -1.0 ("Value") 0.0 ("Value")] -> w224
              tunnel: [255.0 ("Value") 1.0 ("Value") 5.0 ("Value")] -> w223
              tunnel: [128.0 ("Value") 0.0 ("Value") 0.0 ("Value")] -> w222
              tunnel: [64.0 ("Value") 0.5 ("Value") 1.0 ("Value")] -> w221
              frame "PWM" {
              }
              frame "Motor", Default {
              }
              frame "Analog Out" {
              }
            }
            n124 = property on="Motor" class="Clust (strict)"("Visible"=TRUE) -> ()  [unwired: 2 in, 2 out]
            n125 = property on="Value" class="Slide (strict)"("Value"=w222, "Scale.Minimum"=w224, "Scale.Maximum"=w223, "Scale.Increment"=w221) -> ()  [unwired: 2 in, 2 out]
            n126 = property on="On/Off" class="Bool (strict)"("Visible"=w226) -> ()  [unwired: 2 in, 2 out]
            n127 = property on="Test Slider" class="Slide (strict)"("Visible"=w226) -> ()  [unwired: 2 in, 2 out]
            n128 = property on="Test Ring" class="Ring (strict)"("Visible"=w226) -> ()  [unwired: 2 in, 2 out]
            n129 = property on="Rev/Fwd" class="Clust (strict)"("Visible"=w226) -> ()  [unwired: 2 in, 2 out]
          }
          frame "Servo" {
            w242 = FALSE ("Visible")
            n130 = call <vilib>:"NT Read Number.vi"("Name"=w244) -> ("Numeric"=w243:dbl)  [unwired: 9 in, 1 out]
            n131 = property on="Test Slider" class="Slide (strict)"("Visible"=TRUE, "Scale.Maximum"=170.0 ("Scale.Range:Maximum")) -> ()  [unwired: 2 in, 2 out]
            n132 = local write "Test Slider"(w243) -> ()
            n133 = property on="Motor" class="Clust (strict)"("Visible"=w242) -> ()  [unwired: 2 in, 2 out]
            n134 = property on="Rev/Fwd" class="Clust (strict)"("Visible"=w242) -> ()  [unwired: 2 in, 2 out]
            n135 = property on="On/Off" class="Bool (strict)"("Visible"=w242) -> ()  [unwired: 2 in, 2 out]
            n136 = property on="Test Ring" class="Ring (strict)"("Visible"=w242) -> ()  [unwired: 2 in, 2 out]
          }
          frame "Relay", "Solenoid" {
            w245 = FALSE ("Visible")
            n137 = property on="Motor" class="Clust (strict)"("Visible"=w245) -> ()  [unwired: 2 in, 2 out]
            n138 = property on="Test Slider" class="Slide (strict)"("Visible"=w245) -> ()  [unwired: 2 in, 2 out]
            n139 = Search and Replace String(input string=w246, search string="/Value  **", replace string="/Direction") -> (result string=w252:string)  [unwired: 5 in, 3 out]
            n140 = property on="Test Ring" class="Ring (strict)"("Visible"=w245) -> ()  [unwired: 2 in, 2 out]
            n141 = call <vilib>:"NT Read String.vi"("Name"=w252) -> ("String"=w250:string)  [unwired: 9 in, 1 out]
            n142 = Equal?(x="Both directions", y=w250) -> (x = y?=w248:bool)
            n143 = Not(x=w248) -> (.not. x?=w249:bool)
            n144 = property on="Rev/Fwd" class="Clust (strict)"("Visible"=w248) -> ()  [unwired: 2 in, 2 out]
            n145 = property on="On/Off" class="Bool (strict)"("Visible"=w249, "Caption.Text"=w247) -> ()  [unwired: 2 in, 2 out]
          }
          frame "Compressor", "Digital Out" {
            w255 = FALSE ("Visible")
            # "Get direction and finish"
            n146 = property on="Motor" class="Clust (strict)"("Visible"=w255) -> ()  [unwired: 2 in, 2 out]
            n147 = property on="Test Slider" class="Slide (strict)"("Visible"=w255) -> ()  [unwired: 2 in, 2 out]
            n148 = property on="Test Ring" class="Ring (strict)"("Visible"=w255) -> ()  [unwired: 2 in, 2 out]
            n149 = property on="On/Off" class="Bool (strict)"("Visible"=TRUE, "Caption.Text"=w256) -> ()  [unwired: 2 in, 2 out]
            n150 = property on="Rev/Fwd" class="Clust (strict)"("Visible"=FALSE) -> ()  [unwired: 2 in, 2 out]
          }
          frame "Camera" {
            n151 = call <vilib>:"Get Last Path Segment.vi"("String in"=w263) -> ("String out"=w264:string)  [unwired: 10 in]
            n152 = property on="On/Off" class="Bool (strict)"("Visible"=FALSE) -> ()  [unwired: 2 in, 2 out]
            n153 = property on="Motor" class="Clust (strict)"("Visible"=FALSE) -> ()  [unwired: 2 in, 2 out]
            n154 = property on="Rev/Fwd" class="Clust (strict)"("Visible"=FALSE) -> ()  [unwired: 2 in, 2 out]
            n155 = case shown="\"White Balance  **\"" w264 {
              tunnel: w263 -> [w270 w279 w288 w297 w306 _ w312]
              tunnel: w262 -> [w268 w276 w285 w294 w303 _ _]
              frame "Size  **" {
                n156 = Index Array(array=w268) -> (element=w267:cluster{string[]})  [unwired: 1 in]
                n157 = call <vilib>:"NT Read String.vi"("Name"=w270) -> ("String"=w269:string)  [unwired: 9 in, 1 out]
                n158 = Unbundle(w267) -> (w265:string[])
                n159 = Match First String(2:w265, 3:w269) -> (0:w266:i32)  [unwired: 1 out]
                n160 = property on="Test Ring" class="Ring (strict)"("Value"=w266, "Strings []"=w265) -> ()  [unwired: 2 in, 2 out]
                n161 = property on="Test Ring" class="Ring (strict)"("Visible"=TRUE) -> ()  [unwired: 2 in, 2 out]
                n162 = property on="Test Slider" class="Slide (strict)"("Visible"=FALSE) -> ()  [unwired: 2 in, 2 out]
              }
              frame "White Balance  **" {
                n163 = Index Array(array=w276, index=1) -> (element=w277:cluster{string[]})
                n164 = call <vilib>:"NT Read String.vi"("Name"=w279) -> ("String"=w278:string)  [unwired: 9 in, 1 out]
                n165 = Unbundle(w277) -> (w274:string[])
                n166 = Match First String(2:w274, 3:w278) -> (0:w273:i32)  [unwired: 1 out]
                n167 = property on="Test Ring" class="Ring (strict)"("Value"=w273, "Strings []"=w274) -> ()  [unwired: 2 in, 2 out]
                n168 = property on="Test Ring" class="Ring (strict)"("Visible"=TRUE) -> ()  [unwired: 2 in, 2 out]
                n169 = property on="Test Slider" class="Slide (strict)"("Visible"=FALSE) -> ()  [unwired: 2 in, 2 out]
              }
              frame "Exposure  **" {
                n170 = Index Array(array=w285, index=2) -> (element=w286:cluster{string[]})
                n171 = call <vilib>:"NT Read String.vi"("Name"=w288) -> ("String"=w287:string)  [unwired: 9 in, 1 out]
                n172 = Unbundle(w286) -> (w282:string[])
                n173 = Match First String(2:w282, 3:w287) -> (0:w283:i32)  [unwired: 1 out]
                n174 = property on="Test Ring" class="Ring (strict)"("Value"=w283, "Strings []"=w282) -> ()  [unwired: 2 in, 2 out]
                n175 = property on="Test Ring" class="Ring (strict)"("Visible"=TRUE) -> ()  [unwired: 2 in, 2 out]
                n176 = property on="Test Slider" class="Slide (strict)"("Visible"=FALSE) -> ()  [unwired: 2 in, 2 out]
              }
              frame "Exposure Priority  **" {
                n177 = Index Array(array=w294, index=3) -> (element=w295:cluster{string[]})
                n178 = call <vilib>:"NT Read String.vi"("Name"=w297) -> ("String"=w296:string)  [unwired: 9 in, 1 out]
                n179 = Unbundle(w295) -> (w291:string[])
                n180 = Match First String(2:w291, 3:w296) -> (0:w292:i32)  [unwired: 1 out]
                n181 = property on="Test Ring" class="Ring (strict)"("Value"=w292, "Strings []"=w291) -> ()  [unwired: 2 in, 2 out]
                n182 = property on="Test Ring" class="Ring (strict)"("Visible"=TRUE) -> ()  [unwired: 2 in, 2 out]
                n183 = property on="Test Slider" class="Slide (strict)"("Visible"=FALSE) -> ()  [unwired: 2 in, 2 out]
              }
              frame "Color Enable  **" {
                n184 = Index Array(array=w303, index=4) -> (element=w304:cluster{string[]})
                n185 = call <vilib>:"NT Read String.vi"("Name"=w306) -> ("String"=w305:string)  [unwired: 9 in, 1 out]
                n186 = Unbundle(w304) -> (w300:string[])
                n187 = Match First String(2:w300, 3:w305) -> (0:w301:i32)  [unwired: 1 out]
                n188 = property on="Test Ring" class="Ring (strict)"("Value"=w301, "Strings []"=w300) -> ()  [unwired: 2 in, 2 out]
                n189 = property on="Test Ring" class="Ring (strict)"("Visible"=TRUE) -> ()  [unwired: 2 in, 2 out]
                n190 = property on="Test Slider" class="Slide (strict)"("Visible"=FALSE) -> ()  [unwired: 2 in, 2 out]
              }
              frame Default {
                n191 = property on="Test Ring" class="Ring (strict)"("Visible"=FALSE) -> ()  [unwired: 2 in, 2 out]
                n192 = property on="Test Slider" class="Slide (strict)"("Visible"=FALSE) -> ()  [unwired: 2 in, 2 out]
              }
              frame "Brightness  **", "Color Level  **", "Compression  **", "FPS  **", "Sharpness  **" {
                n193 = call <vilib>:"NT Read Number.vi"("Name"=w312) -> ("Numeric"=w311:dbl)  [unwired: 9 in, 1 out]
                n194 = local write "Test Slider"(w311) -> ()
                n195 = property on="Test Slider" class="Slide (strict)"("Visible"=TRUE, "Scale.Maximum"=100.0 ("Scale.Range:Maximum")) -> ()  [unwired: 2 in, 2 out]
                n196 = property on="Test Ring" class="Ring (strict)"("Visible"=FALSE) -> ()  [unwired: 2 in, 2 out]
              }
            }
          }
        }
        n197 = property on="Progress" class="Clust (strict)"("Visible"=FALSE) -> ()  [unwired: 2 in, 2 out]
      }
      event "Test Name": Mouse Enter {
        # "Populate the ring with the list of tests"
        n198 = event-data() -> ()  [unwired: 1 in, 1 out]
        n199 = call <vilib>:"NT Read String Array.vi"("Name"="/TestMode/TestList") -> ("String Array"=w321:string[])  [unwired: 9 in, 1 out]
        n200 = Build Array (concatenate)("Select the test to run...", w321) -> (w320:string[])
        n201 = property on="Test Name" class="Ring (strict)"("Strings []"=w320) -> ()  [unwired: 2 in, 2 out]
      }
      event "Test Name": Value Change {
        w324 = FALSE ("Visible")
        # "Tell the robot the test name to run"
        n202 = event-data() -> ("NewVal"=w328:u16)  [unwired: 1 in]
        n203 = property on="Test Name" class="Ring (strict)"() -> ("Strings []"=w329:string[])  [unwired: 2 in, 2 out]
        n204 = local write "Progress"(T7 {"Test Progress"=0, "Test Progress Text"=""} ("Progress")) -> ()
        n205 = Index Array(array=w329, index=w328) -> (element=w327:string)
        n206 = call <vilib>:"NT Write String.vi"("String"=w327, "Name"="/TestMode/TestName") -> ()  [unwired: 9 in, 1 out]
        n207 = property on="Progress" class="Clust (strict)"("Visible"=TRUE) -> ()  [unwired: 2 in, 2 out]
        n208 = property on="Motor" class="Clust (strict)"("Visible"=w324) -> ()  [unwired: 2 in, 2 out]
        n209 = property on="Test Slider" class="Slide (strict)"("Visible"=w324) -> ()  [unwired: 2 in, 2 out]
        n210 = property on="On/Off" class="Bool (strict)"("Visible"=w324) -> ()  [unwired: 2 in, 2 out]
        n211 = property on="Rev/Fwd" class="Clust (strict)"("Visible"=w324) -> ()  [unwired: 2 in, 2 out]
        n212 = property on="Test Ring" class="Ring (strict)"("Visible"=w324) -> ()  [unwired: 2 in, 2 out]
      }
      event "Command Selection": Value Change {
        # "Get the params and show in table"
        n213 = event-data() -> ("NewVal"=w334:i32)  [unwired: 1 in]
        n214 = property on="Command Selection" class="MCListbox (strict)"() -> ("ItemNames"=w332:string[][])  [unwired: 2 in, 2 out]
        n215 = call <vilib>:"WPI_DashboardUpdate Command Params.vi"("NewVal"=w334, "Commands"=w332, "Param Tbl"=w333) -> ()  [unwired: 8 in, 1 out]
      }
      event "Execute Command": Value Change {
        # "Started one, Unique ID holds\nresponse"
        n216 = event-data() -> ()  [unwired: 1 in, 1 out]
        n217 = property on="Command Selection" class="MCListbox (strict)"() -> ("ItemNames"=w346:string[][])  [unwired: 2 in, 2 out]
        n218 = Index Array(array=w346, index (row)="Command Selection", index (col)=0) -> (element=w344:string)
        n219 = call <vilib>:"Invoke Commands.vi"("Command Params"="Command Params", "Function Name"=w344) -> ("Params"=w340:u8, "Started"=w339:bool)  [unwired: 7 in, 1 out]
        n220 = Array Subset(array="Command Params", length (row)=w340) -> (w341:string[][])  [unwired: 3 in]
        n221 = Select(t="Executing" ("Cmd Status"), s=w339, f="" ("Cmd Status")) -> (s? t:f=→"Cmd Status":string)
      }
      event "Command Selection": Double Click {
        n222 = event-data() -> ("Row"=w356:i32)  [unwired: 1 in]
        n223 = property on="Command Selection" class="MCListbox (strict)"() -> ("ItemNames"=w359:string[][])  [unwired: 2 in, 2 out]
        n224 = local read "Command Params"() -> (w354:string[][])
        n225 = Index Array(array=w359, index (row)=w356, index (col)=0) -> (element=w357:string)
        n226 = call <vilib>:"Invoke Commands.vi"("Command Params"=w354, "Function Name"=w357) -> ("Params"=w353:u8, "Started"=w348:bool)  [unwired: 7 in, 1 out]
        n227 = Array Subset(array=w354, length (row)=w353) -> (w352:string[][])  [unwired: 3 in]
        n228 = Select(t="Executing" ("Cmd Status"), s=w348, f="" ("Cmd Status")) -> (s? t:f=w349:string)
        n229 = local write "Cmd Status"(w349) -> ()
      }
      event "CheckList": Double Click {
        # "Shift clears all"
        # "Update symbols on the listbox"
        n230 = event-data() -> ("PlatMods.Shift"=w362:bool, "Row"=w364:i32)  [unwired: 1 in]
        n231 = case shown="True" w362 {
          tunnel: w364 -> [w368 _]
          tunnel: 1 -> [w367 _]
          frame False {
            n232 = property on="CheckList" class="LstBox (strict)"() -> ("Item Symbols"=w366:i32[])  [unwired: 2 in, 2 out]
            n233 = Replace Array Subset(array=w366, new element=w367, index=w368) -> (w365:i32[])
            n234 = property on="CheckList" class="LstBox (strict)"("Item Symbols"=w365) -> ()  [unwired: 2 in, 2 out]
          }
          frame True {
            w369 = 0 ("Top Row")
            n235 = property on="CheckList" class="LstBox (strict)"() -> ("Number of Rows"=w371:u32)  [unwired: 2 in, 2 out]
            n236 = Initialize Array(0, w371) -> (w370:i32[])
            n237 = property on="CheckList" class="LstBox (strict)"("Top Row"=w369, "Value"=w369, "Item Symbols"=w370) -> ()  [unwired: 2 in, 2 out]
          }
        }
      }
      event "CheckList": Key Down {
        # "Update symbols on the listbox\nLeft and right keys check and uncheck"
        n238 = event-data() -> ("VKey"=w376:T22)  [unwired: 1 in]
        n239 = case shown="\"Left\", \"Right\"" w376 {
          selector: w376 -> [w381 _]
          tunnel: eventvkey."Left" ("VKey") -> [w379 _]
          frame "Left", "Right" {
            n240 = Equal?(x=w379, y=w381) -> (x = y?=w380:bool)
            n241 = Select(t=0, s=w380, f=1) -> (s? t:f=w382:i32)
            n242 = property on="CheckList" class="LstBox (strict)"() -> ("Item Symbols"=w385:i32[])  [unwired: 2 in, 2 out]
            n243 = Replace Array Subset(array=w385, new element=w382, index="CheckList") -> (w384:i32[])
            n244 = property on="CheckList" class="LstBox (strict)"("Item Symbols"=w384) -> ()  [unwired: 2 in, 2 out]
          }
          frame Default {
          }
        }
      }
      event "DB Camera Config": Value Change {
        # "Show or hide the cluster of controls, store in ini file"
        n245 = event-data() -> ("NewVal"=w390:bool)  [unwired: 1 in]
        n246 = case shown="False" w390 {
          tunnel: w389 -> [w399 _]
          tunnel: [w392 w410] -> w388
          tunnel: w387 -> [w391 w410]
          frame False {
            w406 = "Camera"
            w409 = FALSE ("Visible")
            n247 = local read "Camera Settings"() -> (w398:T2)
            n248 = Index Array(array=w399) -> (element=w402:cluster{string[]})  [unwired: 1 in]
            n249 = Unbundle(w398) -> ("Frame Rate"=w397:i32, "Compression"=w396:i32, "Size"=w400:u16)
            n250 = Unbundle(w402) -> (w401:string[])
            n251 = Index Array(array=w401, index=w400) -> (element=w395:string)
            n252 = call-poly <vilib>:"Write Key.vi"("section"=w406, "value"=w395, "key"="Size", "refnum"=w391) -> ("refnum out"=w408:T20)  [unwired: 2 in, 5 out]
            n253 = call-poly <vilib>:"Write Key.vi"("section"=w406, "value"=w397, "key"="FrameRate", "refnum"=w408) -> ("refnum out"=w407:T20)  [unwired: 1 in, 6 out]
            n254 = property on="Camera Settings" class="Clust (strict)"("Visible"=w409) -> ()  [unwired: 2 in, 2 out]
            n255 = local write "DB Camera Config"(w409) -> ()
            n256 = call-poly <vilib>:"Write Key.vi"("section"=w406, "value"=w396, "key"="Compression", "refnum"=w407) -> ("refnum out"=w393:T20)  [unwired: 1 in, 6 out]
            n257 = call <vilib>:"Close Config Data.vi"("refnum"=w393) -> ("file path"=w394:path)  [unwired: 2 in, 8 out]
            n258 = call <vilib>:"Open Config Data.vi"("configuration file path"=w394) -> ("refnum"=w392:T20)  [unwired: 8 in, 2 out]
          }
          frame True {
            n259 = property on="Camera Settings" class="Clust (strict)"("Visible"=TRUE) -> ()  [unwired: 2 in, 2 out]
          }
        }
      }
      event "Camera Settings": Value Change {
        # "Update summary string when any elements of DB camera change"
        n260 = event-data() -> ("NewVal"=w424:T2)  [unwired: 1 in]
        n261 = Index Array(array=w420) -> (element=w419:cluster{string[]})  [unwired: 1 in]
        n262 = Unbundle(w424) -> ("Frame Rate"=w415:i32, "Compression"=w414:i32, "Size"=w417:u16)
        n263 = Unbundle(w419) -> (w418:string[])
        n264 = Index Array(array=w418, index=w417) -> (element=w416:string)
        n265 = Format Into String(format string="%s   %dfps   %d%%", w416, w415, w414) -> (resulting string=w421:string)  [unwired: 2 in, 1 out]
        n266 = Build Array(w421) -> (w422:string[])
        n267 = property on="DB Camera Config" class="Bool (strict)"("Strings [4]"=w422) -> ()  [unwired: 2 in, 2 out]
      }
      event "Motor.Enable": Value Change {
        # "When the test mode otor enable helper is set, update that\ntree row item's value"
        n268 = event-data() -> ("NewVal"=w431:bool)  [unwired: 1 in]
        n269 = Unbundle("Motor") -> ("Value"=w430:dbl)  [unwired: 1 out]
        n270 = Select(t=w430, s=w431, f=0.0) -> (s? t:f=w428:dbl)
        n271 = call <vilib>:"NT Write Number.vi"("Numeric"=w428, "Name"=w427) -> ()  [unwired: 9 in, 1 out]
      }
      event "Test Slider": Value Change {
        # "When the test mode slider helper is set, update that\ntree row item's value"
        n272 = event-data() -> ("NewVal"=w435:dbl)  [unwired: 1 in]
        n273 = call <vilib>:"NT Write Number.vi"("Numeric"=w435, "Name"=w436) -> ()  [unwired: 9 in, 1 out]
      }
      event "On/Off": Value Change {
        # "When the test mode on/off helper value is set, update that\ntree row item's value"
        n274 = event-data() -> ("NewVal"=w441:bool)  [unwired: 1 in]
        n275 = Boolean To (0,1)(Boolean=w441) -> (0, 1=w440:i16)
        n276 = call <vilib>:"NT Write Number.vi"("Numeric"=w440, "Name"=w439) -> ()  [unwired: 9 in, 1 out]
      }
      event "Rev/Fwd": Value Change {
        # "When the test mode helper value for relays is set, update that\ntree row item's value"
        n277 = event-data() -> ("NewVal.Forward"=w450:bool, "NewVal.Reverse"=w449:bool)  [unwired: 1 in]
        n278 = Boolean To (0,1)(Boolean=w450) -> (0, 1=w446:i16)
        n279 = Boolean To (0,1)(Boolean=w449) -> (0, 1=w448:i16)
        n280 = Negate(x=w448) -> (-x=w447:i16)
        n281 = Add(x=w446, y=w447) -> (x+y=w445:i16)
        n282 = call <vilib>:"NT Write Number.vi"("Numeric"=w445, "Name"=w444) -> ()  [unwired: 9 in, 1 out]
      }
      event "Test Ring": Value Change {
        # "When a test mode helper value is selected from the ring,\nset the tree item's variable to the string value"
        n283 = event-data() -> ("NewVal"=w455:u16)  [unwired: 1 in]
        n284 = property on="Test Ring" class="Ring (strict)"() -> ("Strings []"=w456:string[])  [unwired: 2 in, 2 out]
        n285 = Index Array(array=w456, index=w455) -> (element=w454:string)
        n286 = call <vilib>:"NT Write String.vi"("String"=w454, "Name"=w453) -> ()  [unwired: 9 in, 1 out]
      }
      event "Rec Mode": Value Change {
        # "Update globals for recording mode and path to read log from.\nClear when logging and let NetworkTables set path for vision to\nuse."
        n287 = event-data() -> ("NewVal"=w468:enum32{"Stop", "Record", "Playback"})  [unwired: 1 in]
        n288 = global write "WPI_DashboardLogging Global.vi" "Logging Filename"(path "") -> ()
        n289 = global write "WPI_DashboardLogging Global.vi" "Recording"(w468) -> ()
        n290 = case shown="\"Playback\"" w468 {
          tunnel: w467 -> [_ w470 w479]
          tunnel: [_ _ w478] -> w464
          tunnel: [_ _ w477] -> _
          tunnel: w462 -> [_ _ w475]
          tunnel: cluster{i32, i32} {-250, 170} -> [_ _ w474]
          tunnel: [_ _ T23 {"Image Size"=TRUE, "Image Type"=TRUE, "Pixel Value"=TRUE, "ROI Information"=TRUE, "Zoom Factor"=FALSE} ("Image Information Shown:All Elements")] -> w460
          tunnel: [_ _ TRUE ("Zoom Factor")] -> w459
          tunnel: w458 -> [_ _ w471]
          frame Default {
          }
          frame "Stop", "Record" {
            # "Place Window too"
            n291 = invoke class="VI" method="FP.Close"(reference=w470) -> (reference out=w469:refnum<vi>)  [unwired: 2 in, 2 out]
            n292 = invoke class="VI" method="Abort VI"(reference=w469) -> ()  [unwired: 2 in, 3 out]
          }
          frame "Playback" {
            n293 = call "Open Playback Panel.vi"("Offset"=w474, "DB VI Ref"=w475, "Playback in"=w479) -> ("Playback out"=w476:refnum<vi>)  [unwired: 8 in]
            n294 = register-events(w476, w471) -> (reference out=w478:refnum<event-registration>, error out=w477:errorcluster)  [unwired: 2 in]
          }
        }
        n295 = property on="Camera Image" class="ImageControl"("Image Information Shown"=w460, "Image Information Visible"=w459) -> ()  [unwired: 2 in, 2 out]
        n296 = call <vilib>:"WPI_DashboardNT Log FieldName Cache.vi"("Operation"=enum16{"Lookup/Add", "Index", "Clear"}."Clear") -> ()  [unwired: 8 in, 3 out]
      }
      event Panel Close {
        w481 = enum32{"Stop", "Record", "Playback"}."Stop" ("Rec Mode")
        # "Playback window has been closed, abort"
        n297 = event-data() -> ()  [unwired: 1 in, 4 out]
        n298 = local write "Rec Mode"(w481) -> ()
        n299 = global write "WPI_DashboardLogging Global.vi" "Recording"(w481) -> ()
      }
      event Panel Close {
        # "Abort playback window and ourself"
        n300 = event-data() -> ()  [unwired: 1 in, 4 out]
        n301 = invoke class="VI" method="FP.Close"(reference=w487) -> (reference out=w486:refnum<vi>)  [unwired: 2 in, 2 out]
        n302 = invoke class="VI" method="Abort VI"(reference=w486) -> (error out=w485:errorcluster)  [unwired: 2 in, 2 out]
        n303 = invoke class="VI" method="Abort VI"(error in=w485) -> ()  [unwired: 2 in, 3 out]
      }
      event User Event {
        n304 = event-data() -> ("IDs"=w495:cluster{"RPC field ID":u16, "Unique ID":u16}, "String"=w494:string)  [unwired: 1 in]
        n305 = Bundle("IDs"=w495, "String"=w494) -> (w493:T9)  [unwired: 1 in]
        n306 = call <vilib>:"Retrieve RPC Response.vi"("RPC Response"=w493) -> ("Output"=w490:string[][])  [unwired: 10 in]
        n307 = Build Array (concatenate)(w488, w490) -> (w489:string[][])
        n308 = local write "Command Params"(w489) -> ()
        n309 = local write "Cmd Status"("" ("Cmd Status")) -> ()
      }
      event "Vision": Value Change {
        # "Enable/Disable Compression slider.\nHW USB is hard-coded into the camera"
        n310 = event-data() -> ("NewVal"=w502:u16)  [unwired: 1 in]
        n311 = Equal?(x=w502, y=u32 2 ("milliseconds to wait")) -> (x = y?=w500:bool)
        n312 = Select(t=T24."Disabled and Grayed Out" ("Disabled"), s=w500, f=T24."Enabled" ("Disabled")) -> (s? t:f=w497:T24)
        n313 = property on="Compression" class="Slide (strict)"("DisabledEnum"=w497) -> ()  [unwired: 2 in, 2 out]
      }
    }
  }
  n314 = while {
    tunnel: w47 -> [w505]
    i -> [w508]
    stop <- FALSE stop-if-true
    n315 = Wait (ms)(milliseconds to wait=u32 100) -> ()  [unwired: 1 out]
    n316 = case shown="\"Playback\"" "Rec Mode" {
      tunnel: w508 -> [_ _ w523]
      tunnel: [u32 2829099 ("Base Color") u32 11141120 ("Target Color") w512] -> w504
      frame "Stop", Default {
        # "Reset the color, extra updates don't cost much"
      }
      frame "Record" {
      }
      frame "Playback" {
        # "Playback"
        n317 = Quotient & Remainder(x=w523, y=u32 50 ("milliseconds to wait")) -> (x-y*floor(x/y)=w519:u32)  [unwired: 1 out]
        n318 = Divide(x=w519, y=u32 50 ("milliseconds to wait")) -> (x/y=w516:dbl)
        n319 = Multiply(x=6.283185307179586, y=w516) -> (x*y=w521:dbl)
        n320 = Sine(x=w521) -> (sin(x)=w520:dbl)
        n321 = Absolute Value(x=w520) -> (abs(x)=w513:dbl)
        n322 = call "Interpolate RGB Color.vi"("Proportion"=w513, "Target Color"=u32 30976, "Base Color"=u32 2829099) -> ("Result Color"=w512:u32)  [unwired: 8 in]
      }
    }
    n323 = property class="Pane"(reference=w505, "PaneColor"=w504) -> ()  [unwired: 1 in, 2 out]
  }
  n324 = local write "Dashboard Tab"(T1."Drive" ("Dashboard Tab")) -> ()
  n325 = property on="On/Off" class="Bool (strict)"("Visible"=w15) -> ()  [unwired: 2 in, 2 out]
  n326 = property on="Motor" class="Clust (strict)"("Visible"=w15) -> ()  [unwired: 2 in, 2 out]
  n327 = property on="Progress" class="Clust (strict)"("Visible"=w15) -> ()  [unwired: 2 in, 2 out]
  n328 = property on="Test Ring" class="Ring (strict)"("Visible"=w15) -> ()  [unwired: 2 in, 2 out]
  n329 = property on="Rev/Fwd" class="Clust (strict)"("Visible"=w15) -> ()  [unwired: 2 in, 2 out]
  n330 = property on="Camera Settings" class="Clust (strict)"("Visible"=w15) -> ()  [unwired: 2 in, 2 out]
  n331 = while {
    tunnel: u16 1741 ("timeout ms (25000)") -> [w525]
    stop <- FALSE stop-if-true
    n332 = TCP Create Listener(10:w525) -> (0:w524:errorcluster, 3:w526:refnum<k5>)  [unwired: 4 in, 1 out]
    n333 = case shown="No Error" w524 {
      selector: w524 -> [w528 _]
      tunnel: w526 -> [w529 _]
      frame No Error {
        n334 = while {
          tunnel: w529 -> [w532]
          tunnel: w528 -> [w531]
          stop <- FALSE stop-if-true
          n335 = TCP Wait On Listener(8:w531, 11:w532) -> (0:w533:errorcluster, 4:w534:refnum<k5>)  [unwired: 2 in, 3 out]
          n336 = local write "TCP"(w534) -> ()
          n337 = case shown="No Error" w533 {
            frame No Error {
            }
            frame Error {
              n338 = Wait (ms)(milliseconds to wait=u32 1000) -> ()  [unwired: 1 out]
            }
          }
        }
      }
      frame Error {
        n339 = Wait (ms)(milliseconds to wait=u32 1000) -> ()  [unwired: 1 out]
      }
    }
  }
  n340 = local write "DB Camera Config"(w15) -> ()
  n341 = local write "Command Params"(string[][] [] ("Command Params")) -> ()
  n342 = global write "WPI_DashboardLogging Global.vi" "Recording"(w41) -> ()
  n343 = local write "Command Selection"(u16 0 ("milliseconds to wait")) -> ()
  n344 = local write "Rec Mode"(w41) -> ()
